vi "getIrf (SubVI).vi"(8 "error in":errorcluster, 10 "CtrlV":dbl, 11 "APD":T1) -> (0 "error out":errorcluster, 2 "irfTNorm":dbl[](array[numeric]), 3 "irfIdx":i32)   [LabVIEW 2020]
uses:
  APD.ctl
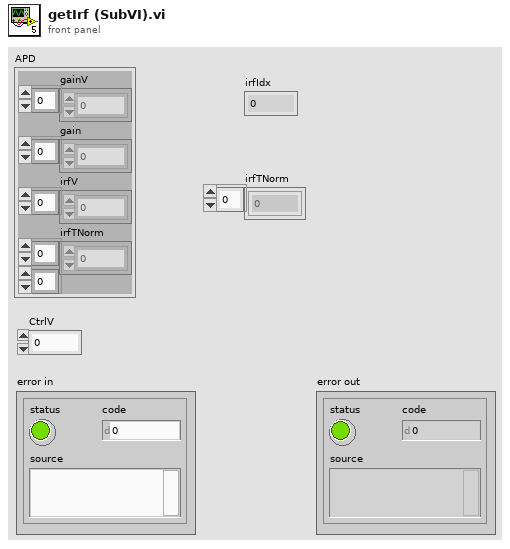
[diagram p1: front panel]
types:
  T1 = typedef "APD.ctl" = cluster{"gainV":dbl[], "gain":dbl[], "irfV":dbl[], "irfTNorm":dbl[][]}
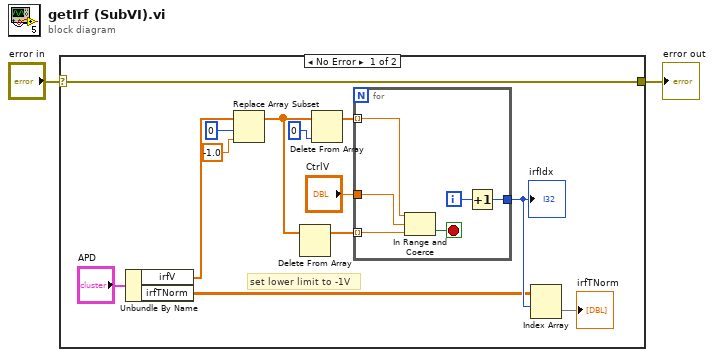
[diagram p0: block diagram]
diagram:
  n1 = case shown="No Error" "error in" {
    selector: "error in" -> [w3 w22]
    tunnel: [w3 w22] -> w1
    frame No Error {
      # "set lower limit to -1V"
      n2 = Unbundle By Name("APD") -> ("irfV"=w9:dbl[], "irfTNorm"=w13:dbl[][])
      n3 = Replace Array Subset(array=w9, new element=-1.0 ("new element/subarray"), index=0) -> (w12:dbl[])
      n4 = Delete From Array(array=w12) -> (array with subset deleted=w6:dbl[])  [unwired: 2 in, 1 out]
      n5 = Delete From Array(array=w12, index=0) -> (array with subset deleted=w7:dbl[])  [unwired: 1 in, 1 out]
      n6 = for {
        tunnel: w6 -> [w21] mode=indexing
        tunnel: w7 -> [w20] mode=indexing
        tunnel: "CtrlV" -> [w19]
        tunnel: [w17] -> w14
        i -> [w18]
        stop <- w16 stop-if-true
        n7 = In Range and Coerce(upper limit=w20, x=w19, lower limit=w21) -> (In Range?=w16:bool)  [unwired: 1 out]
        n8 = Increment(x=w18) -> (x+1=w17:i32)
      }
      "irfIdx" <- w14
      n9 = Index Array(array=w13, index (row)=w14) -> (element=→"irfTNorm":dbl[])  [unwired: 1 in]
    }
    frame Error {
    }
  }
  "error out" <- w1
